vi "VINeedTest.vi"(8 "error in":errorcluster, 10 "b":dbl, 11 "a":dbl) -> (0 "error out":errorcluster, 3 "c":dbl)   [LabVIEW 2019, in "UnitTestFramework.lvclass"]
uses:
  UnitTestFramework.lvclass
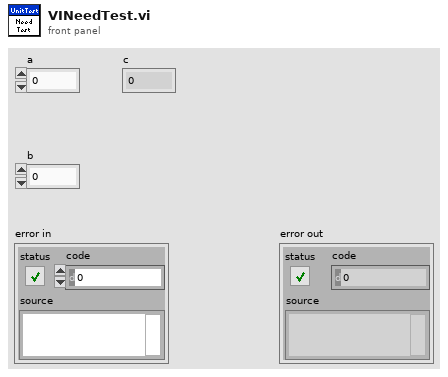
[diagram p1: front panel]
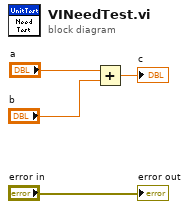
[diagram p0: block diagram]
diagram:
  n1 = Add(x="a", y="b") -> (x+y=→"c":dbl)
  "error out" <- "error in"
